vi "PID MeaNoise.vi"(2 "OK":bool, 3 "PV %":dbl format="%.2f") -> (1 "Noise":dbl format="%.2f")   [LabVIEW 2020, in "NI_PID_autopid.lvlib"]
doc: "This VI calculates the root mean square of the sampled process variable. This value is used as an estimate of the noise on the process variable."
uses:
  <vilib>/addons/control/pid/NI_PID_autopid.lvlib
panel:
  # "Measure Process Noise"
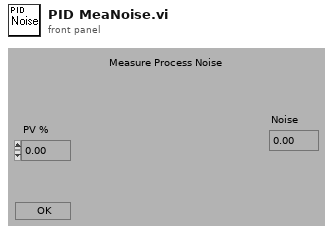
[diagram p1: front panel]
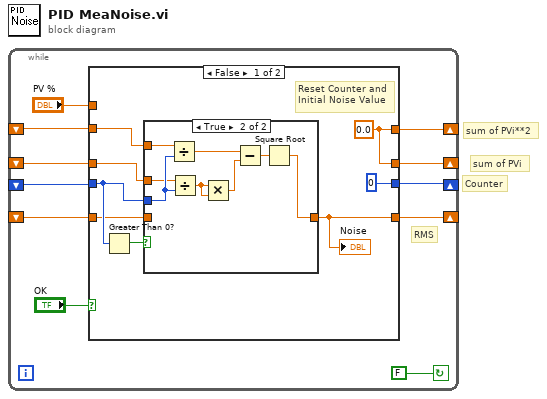
[diagram p0: block diagram]
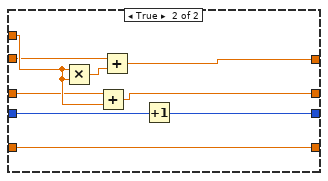
[diagram p3: hidden frame]
diagram:
  # "sum of PVi"
  # "sum of PVi**2"
  # "Counter"
  n1 = while {
    shift-left: _ -> [w2]
    shift-right: [w3] -> _
    shift-left: _ -> [w5]
    shift-right: [w4] -> _
    shift-left: _ -> [w8]
    shift-right: [w9] -> _
    shift-left: _ -> [w10]
    shift-right: [w11] -> _
    stop <- FALSE continue-if-true
    # "RMS"
    n2 = case shown="False" "OK" {
      tunnel: "PV %" -> [_ w37]
      tunnel: w8 -> [w15 w36]
      tunnel: [0 w29] -> w9
      tunnel: [w18 w35] -> w11
      tunnel: w10 -> [w16 w34]
      tunnel: w5 -> [w17 w33]
      tunnel: [w18 w32] -> w4
      tunnel: [w12 w31] -> w3
      tunnel: w2 -> [w13 w31]
      frame False {
        w18 = 0.0
        # "Reset Counter and\nInitial Noise Value"
        n3 = Greater Than 0?(x=w15) -> (x > 0?=w14:bool)
        n4 = case shown="True" w14 {
          tunnel: w15 -> [_ w23]
          tunnel: w16 -> [_ w22]
          tunnel: w17 -> [_ w21]
          tunnel: [w20 w28] -> w12
          tunnel: w13 -> [w20 _]
          frame False {
          }
          frame True {
            n5 = Divide(x=w22, y=w23) -> (x/y=w25:dbl)
            n6 = Divide(x=w21, y=w23) -> (x/y=w24:dbl)
            n7 = Multiply(x=w24, y=w24) -> (x*y=w26:dbl)
            n8 = Subtract(x=w25, y=w26) -> (x-y=w27:dbl)
            n9 = Square Root(x=w27) -> (sqrt(x)=w28:dbl)
          }
        }
        "Noise" <- w12
      }
      frame True {
        n10 = Multiply(x=w37, y=w37) -> (x*y=w30:dbl)
        n11 = Add(x=w33, y=w37) -> (x+y=w32:dbl)
        n12 = Add(x=w34, y=w30) -> (x+y=w35:dbl)
        n13 = Increment(x=w36) -> (x+1=w29:i32)
      }
    }
  }
